vi "processesAbsorptionImageNEW.vi"(8 "error in (no error)":errorcluster, 10 "ImagePaths in":path[](array[path])) -> (0 "error out":errorcluster, 1 "number":dbl, 2 "ImagePaths out":path[](array[path]), 3 "BECImageProcessor out":refnum<class "BECImageProcessor.lvclass">, 4 "width":dbl)   [LabVIEW 2009, in "Tools.lvlib" / "Imaging.lvlib" / "BECImageProcessor.lvclass"]
uses:
  BECImageProcessor.lvclass
  <vilib>/vision/NI_Vision_Development_Module.lvlib
  Filing.lvlib
  Filing/FileNeologist/FileNeologist.lvclass
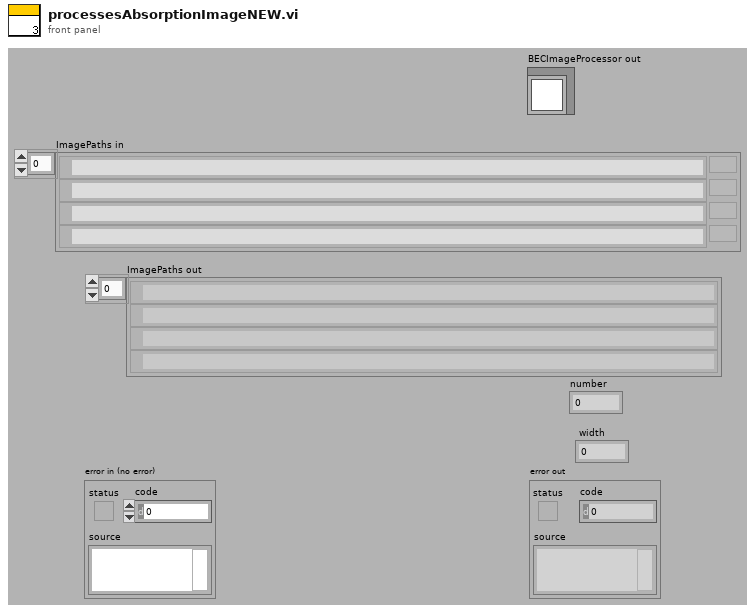
[diagram p1: front panel]
types:
  T1 = typedef "Image Type" = u32
  T2 = typedef "IMAQ Image.ctl" = refnum<image>
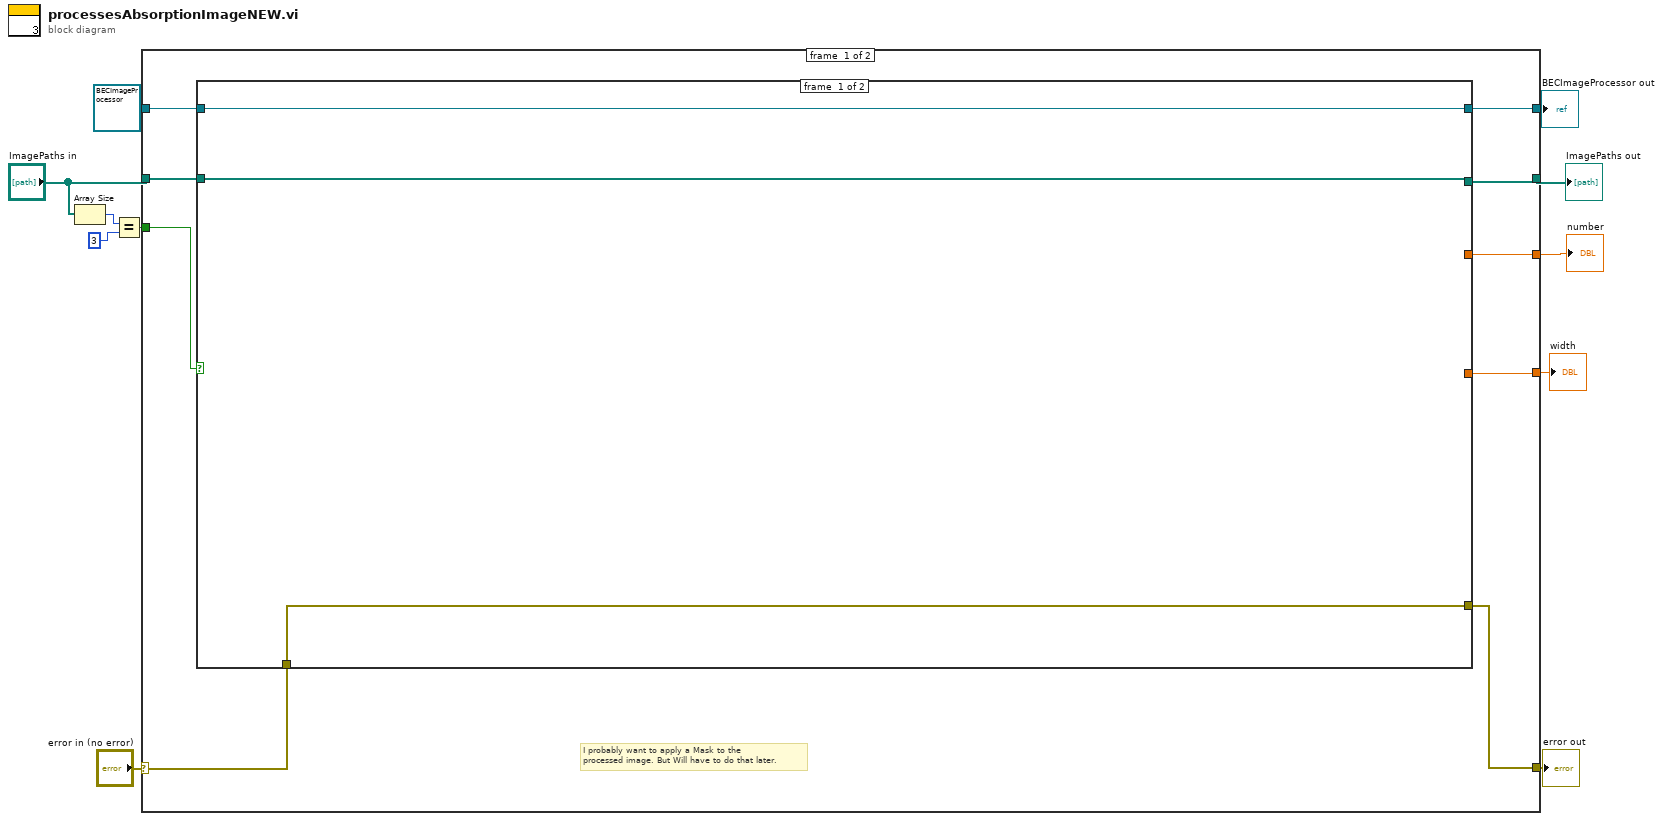
[diagram p0: block diagram]
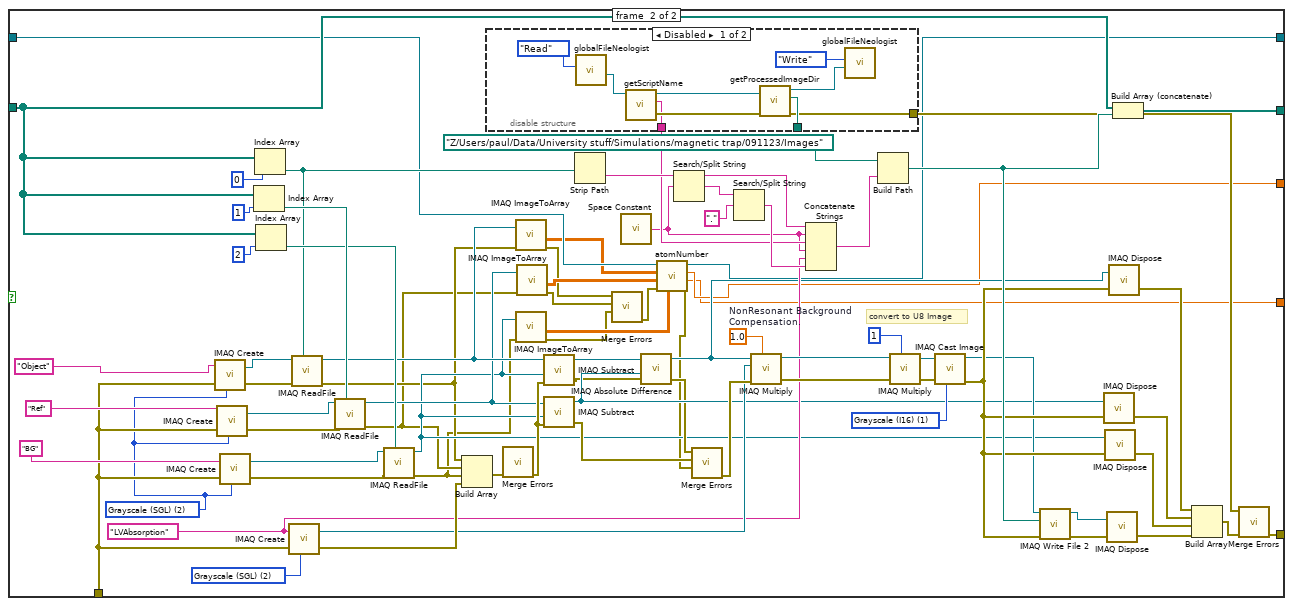
[diagram p2: hidden frame]
diagram:
  n1 = Array Size(array="ImagePaths in") -> (size(s)=w5:i32)
  n2 = Equal?(x=w5, y=3) -> (x = y?=w3:bool)
  n3 = case shown="No Error" "error in (no error)" {
    selector: "error in (no error)" -> [w20 w112]
    tunnel: [w17 w112] -> w8
    tunnel: [w14 w111] -> w10
    tunnel: refnum<class "BECImageProcessor.lvclass"> refnum ("BECImageProcessor in") -> [w15 w111]
    tunnel: "ImagePaths in" -> [w19 _]
    tunnel: [w18 _] -> w9
    tunnel: w3 -> [w16 _]
    tunnel: [w13 _] -> w2
    tunnel: [w12 _] -> w1
    frame #0 {
      # "I probably want to apply a Mask to the\nprocessed image. But Will have to do that later."
      n4 = case shown="True" w16 {
        tunnel: w20 -> [w22 w94]
        tunnel: w19 -> [w23 w38]
        tunnel: [w23 w81] -> w18
        tunnel: [w22 w72] -> w17
        tunnel: w15 -> [w21 w37]
        tunnel: [w21 w29] -> w14
        tunnel: [_ w28] -> w13
        tunnel: [_ w27] -> w12
        frame #0 {
        }
        frame #1 {
          w61 = T1 1 items=["Grayscale (U8)", "Grayscale (I16)", "Grayscale (SGL)", "Complex (CSG)", "RGB (U32)", "HSL (U32)", "RGB (U64)"] ("Image Type")
          w63 = T1 2 items=["Grayscale (U8)", "Grayscale (I16)", "Grayscale (SGL)", "Complex (CSG)", "RGB (U32)", "HSL (U32)", "RGB (U64)"] ("Image Type")
          w71 = T1 2 items=["Grayscale (U8)", "Grayscale (I16)", "Grayscale (SGL)", "Complex (CSG)", "RGB (U32)", "HSL (U32)", "RGB (U64)"] ("Image Type")
          w59 = 1.0  # NonResonant Background Compensation.
          w50 = "LVAbsorption"
          # "convert to U8 Image"
          n5 = call "IMAQ Create"("Image Name"="Object", "Image Type"=w63, "error in (no error)"=w94) -> ("New Image"=w64:T2, "error out"=w69:errorcluster)  [unwired: 2 in]
          n6 = call "IMAQ Create"("Image Name"="Ref", "Image Type"=w63, "error in (no error)"=w94) -> ("New Image"=w68:T2, "error out"=w67:errorcluster)  [unwired: 2 in]
          n7 = call "IMAQ Create"("Image Name"="BG", "Image Type"=w63, "error in (no error)"=w94) -> ("New Image"=w66:T2, "error out"=w65:errorcluster)  [unwired: 2 in]
          n8 = Index Array(array=w38, index=1) -> (element=w96:path)
          n9 = Index Array(array=w38, index=0) -> (element=w88:path)
          n10 = Index Array(array=w38, index=2) -> (element=w95:path)
          n11 = call "IMAQ Create"("Image Name"=w50, "Image Type"=w71, "error in (no error)"=w94) -> ("New Image"=w89:T2, "error out"=w93:errorcluster)  [unwired: 2 in]
          n12 = call "IMAQ ReadFile"("File Path"=w88, "error in (no error)"=w69, "Image"=w64) -> ("error out"=w39:errorcluster, "Image Out"=w42:T2)  [unwired: 4 in, 3 out]
          n13 = call "IMAQ ReadFile"("File Path"=w96, "error in (no error)"=w67, "Image"=w68) -> ("error out"=w25:errorcluster, "Image Out"=w41:T2)  [unwired: 4 in, 3 out]
          n14 = call "IMAQ ReadFile"("File Path"=w95, "error in (no error)"=w65, "Image"=w66) -> ("error out"=w24:errorcluster, "Image Out"=w40:T2)  [unwired: 4 in, 3 out]
          n15 = Build Array(w39, w25, w24, w93) -> (w92:errorcluster[])
          n16 = disable-structure shown="Disabled" {
            disable-tunnel: [w109 _] -> _
            disable-tunnel: [w106 _] -> w53
            disable-tunnel: [w102 _] -> w51
            frame #0 {
              n17 = call "globalFileNeologist.vi"("Action"=enum16{"Write", "Read"}."Read") -> ("FileNeologist out"=w103:refnum<class "FileNeologist.lvclass">)  [unwired: 10 in]
              n18 = call-dynamic "getScriptName.vi"("FileNeologist.lvclass in"=w103) -> ("error out"=w104:errorcluster, "scriptName"=w102:string, "FileNeologist.lvclass out"=w105:refnum<class "FileNeologist.lvclass">)  [unwired: 8 in]
              n19 = call-dynamic "getProcessedImageDir.vi"("error in (no error)"=w104, "FileNeologist in"=w105) -> ("error out"=w106:errorcluster, "Path"=w109:path, "FileNeologist out"=w108:refnum<class "FileNeologist.lvclass">)  [unwired: 7 in]
              n20 = call "globalFileNeologist.vi"("FileNeologist in"=w108, "Action"=enum16{"Write", "Read"}."Write") -> ()  [unwired: 9 in, 1 out]
            }
            frame #1 {
            }
          }
          n21 = call <vilib>:"Merge Errors.vi"("error array in"=w92) -> ("error out"=w91:errorcluster)  [unwired: 6 in]
          n22 = call "IMAQ ImageToArray"("error in (no error)"=w39, "Image"=w42) -> ("Image Pixels (Float)"=w36:sgl[][], "error out"=w33:errorcluster)  [unwired: 2 in, 3 out]
          n23 = call "IMAQ ImageToArray"("error in (no error)"=w24, "Image"=w40) -> ("Image Pixels (Float)"=w34:sgl[][], "error out"=w31:errorcluster)  [unwired: 2 in, 3 out]
          n24 = call "IMAQ ImageToArray"("error in (no error)"=w25, "Image"=w41) -> ("Image Pixels (Float)"=w35:sgl[][], "error out"=w32:errorcluster)  [unwired: 2 in, 3 out]
          n25 = call "IMAQ Subtract"("Image Src A"=w42, "Image Src B"=w40, "error in (no error)"=w91) -> ("Image Dst Out"=w47:T2, "error out"=w44:errorcluster)  [unwired: 4 in]
          n26 = call "IMAQ Subtract"("Image Src A"=w41, "Image Src B"=w40, "error in (no error)"=w91) -> ("Image Dst Out"=w46:T2, "error out"=w70:errorcluster)  [unwired: 4 in]
          n27 = Strip Path(path=w88) -> (name=w86:string)  [unwired: 1 out]
          n28 = call <vilib>:"Merge Errors.vi"("error in 3 (no error)"=w31, "error in 2 (no error)"=w32, "error in 1 (no error)"=w33) -> ("error out"=w30:errorcluster)  [unwired: 4 in]
          n29 = call <vilib>:"Space Constant.vi"() -> ("String"=w49:string)
          n30 = call "IMAQ Absolute Difference"("Image Src A"=w47, "Image Src B"=w46, "error in (no error)"=w44) -> ("Image Dst Out"=w45:T2, "error out"=w43:errorcluster)  [unwired: 4 in]
          n31 = call "atomNumber.vi"("Image bg"=w34, "error in (no error)"=w30, "Image ref"=w35, "Image object"=w36, "BECImageProcessor in"=w37) -> ("error out"=w26:errorcluster, "x width"=w27:dbl, "number"=w28:dbl, "BECImageProcessor out"=w29:refnum<class "BECImageProcessor.lvclass">)  [unwired: 1 in, 2 out]
          n32 = Search/Split String(string=w86, search string/char (-)=w49) -> (substring before match=w84:string, match + rest of string=w85:string)  [unwired: 1 in, 1 out]
          n33 = call <vilib>:"Merge Errors.vi"("error in 3 (no error)"=w26, "error in 2 (no error)"=w70, "error in 1 (no error)"=w43) -> ("error out"=w90:errorcluster)  [unwired: 4 in]
          n34 = Search/Split String(string=w85, search string/char (-)=".") -> (match + rest of string=w83:string)  [unwired: 1 in, 2 out]
          n35 = call "IMAQ Multiply"("Image Src A"=w45, "Constant"=w59, "Image Dst"=w89, "error in (no error)"=w90) -> ("Image Dst Out"=w58:T2, "error out"=w57:errorcluster)  [unwired: 3 in]
          n36 = Concatenate Strings(w84, w49, w51, w49, w50, w83) -> (w82:string)
          n37 = Build Path(base path=path "Z:/Users/paul/Data/University stuff/Simulations/magnetic trap/091123/Images", name or relative path=w82) -> (appended path=w80:path)
          n38 = call "IMAQ Multiply"("Image Src A"=w58, "Constant"=1, "error in (no error)"=w57) -> ("Image Dst Out"=w54:T2, "error out"=w55:errorcluster)  [unwired: 4 in]
          n39 = call "IMAQ Cast Image"("Image Type"=w61, "error in (no error)"=w55, "Image Src"=w54) -> ("error out"=w62:errorcluster, "Image Dst Out"=w60:T2)  [unwired: 7 in]
          n40 = call-poly "IMAQ Write File 2"("error in (no error)"=w62, "File Path"=w80, "Image"=w60) -> ("error out"=w78:errorcluster, "Image Out (duplicate)"=w79:T2)  [unwired: 7 in]
          n41 = call "IMAQ Dispose"("Image"=w46, "error in (no error)"=w62) -> ("error out"=w76:errorcluster)  [unwired: 4 in]
          n42 = call "IMAQ Dispose"("Image"=w40, "error in (no error)"=w62) -> ("error out"=w75:errorcluster)  [unwired: 4 in]
          n43 = call "IMAQ Dispose"("Image"=w79, "error in (no error)"=w78) -> ("error out"=w74:errorcluster)  [unwired: 4 in]
          n44 = call "IMAQ Dispose"("Image"=w45, "error in (no error)"=w62) -> ("error out"=w77:errorcluster)  [unwired: 4 in]
          n45 = Build Array (concatenate)(w38, w80) -> (w81:path[])
          n46 = Build Array(w77, w76, w75, w74) -> (w73:errorcluster[])
          n47 = call <vilib>:"Merge Errors.vi"("error array in"=w73, "error in 1 (no error)"=w53) -> ("error out"=w72:errorcluster)  [unwired: 5 in]
        }
      }
    }
    frame #1 {
    }
  }
  "error out" <- w8
  "BECImageProcessor out" <- w10
  "ImagePaths out" <- w9
  "number" <- w2
  "width" <- w1
